vi "Remove Duplicates from 1D String Array.vi"(11 "Input Array":string[](array[string])) -> (3 "Output Array":string[](array[string]))   [LabVIEW 2014]
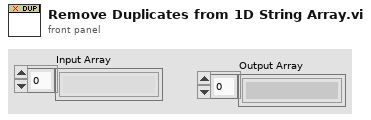
[diagram p1: front panel]
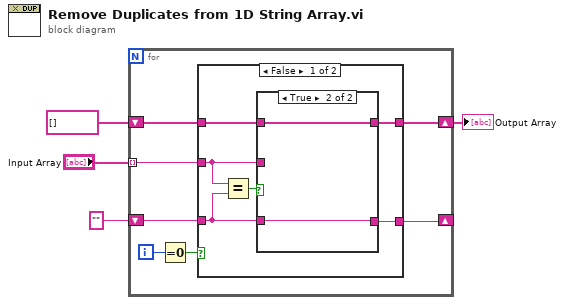
[diagram p0: block diagram]
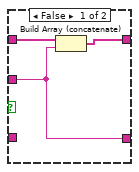
[diagram p2: hidden frame]
diagram:
  n1 = for {
    tunnel: "Input Array" -> [w9] mode=indexing
    shift-right: [w7] -> _
    shift-left: "" -> [w8]
    shift-right: [w5] -> w1
    shift-left: string[] [] -> [w6]
    i -> [w11]
    n2 = Equal To 0?(x=w11) -> (x = 0?=w10:bool)
    n3 = case shown="False" w10 {
      tunnel: w9 -> [w14 w23]
      tunnel: w8 -> [w16 _]
      tunnel: [w15 w23] -> w7
      tunnel: w6 -> [w13 w24]
      tunnel: [w12 w24] -> w5
      frame False {
        n4 = Equal?(x=w14, y=w16) -> (x = y?=w17:bool)
        n5 = case shown="True" w17 {
          tunnel: [w19 w22] -> w15
          tunnel: w16 -> [_ w22]
          tunnel: w14 -> [w19 _]
          tunnel: w13 -> [w20 w21]
          tunnel: [w18 w21] -> w12
          frame False {
            n6 = Build Array (concatenate)(w20, w19) -> (w18:string[])
          }
          frame True {
          }
        }
      }
      frame True {
      }
    }
  }
  "Output Array" <- w1
